vi "Validation Class.vi"() -> ()   [LabVIEW 2020, in "Library Instrument & Equipement.lvlib" / "Library FireBase.lvlib" / "Firebase Recovery_SN.lvclass"]
uses:
  Firebase Recovery_SN.lvclass
  C:/Users/ngarcin/OneDrive - Altyor/Standard TB/Class/Firebase/Source/Firebase Driver/Firebase Driver.lvclass
  Firebase Recovery_SN.lvclass/Firebase Recovery_SN.ctl
panel:
  out "PN":string
  out "Format_SN":string
  out "Incremental_Number":string
  out "sortie d'erreur":errorcluster
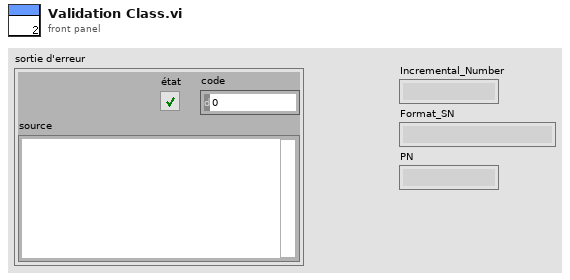
[diagram p1: front panel]
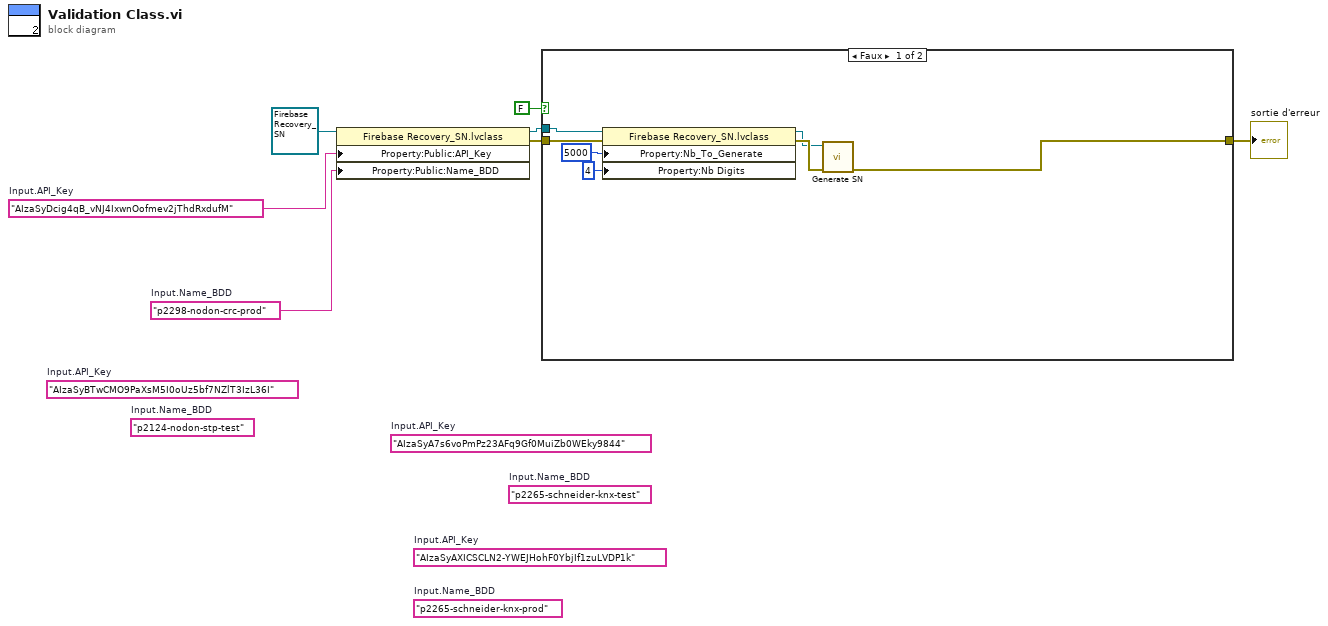
[diagram p0: block diagram]
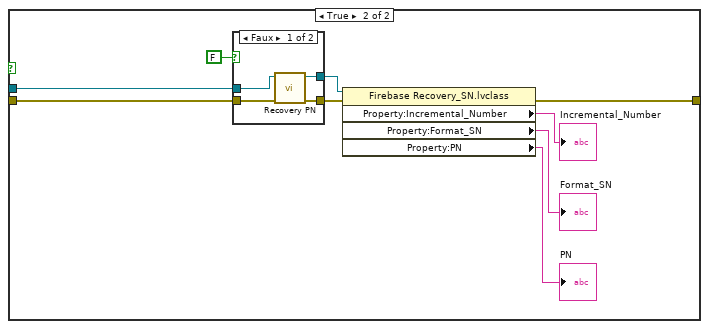
[diagram p2: hidden frame]
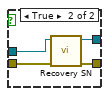
[diagram p3: hidden frame]
diagram:
  (unwired) "AIzaSyBTwCMO9PaXsM5I0oUz5bf7NZlT3IzL36I"  # Input.API_Key
  (unwired) "p2124-nodon-stp-test"  # Input.Name_BDD
  (unwired) "AIzaSyA7s6voPmPz23AFq9Gf0MuiZb0WEky9844"  # Input.API_Key
  (unwired) "p2265-schneider-knx-test"  # Input.Name_BDD
  w2 = "AIzaSyDcig4qB_vNJ4IxwnOofmev2jThdRxdufM"  # Input.API_Key
  w1 = "p2298-nodon-crc-prod"  # Input.Name_BDD
  (unwired) "AIzaSyAXICSCLN2-YWEJHohF0YbjIf1zuLVDP1k"  # Input.API_Key
  (unwired) "p2265-schneider-knx-prod"  # Input.Name_BDD
  n1 = property class="Firebase Recovery_SN.lvclass"(reference=refnum<class "Firebase Recovery_SN.lvclass"> refnum ("Build Library FireBase.lvlib:Firebase AssembledProducts.lvclass"), "Property:Public:API_Key"=w2, "Property:Public:Name_BDD"=w1) -> (reference out=w6:refnum<class "Firebase Recovery_SN.lvclass">, error out=w5:errorcluster)  [unwired: 1 in]
  n2 = case shown="Faux" FALSE {
    tunnel: w6 -> [w11 w23]
    tunnel: w5 -> [w13 w22]
    tunnel: [w14 w19] -> w4
    frame False {
      n3 = property class="Firebase Recovery_SN.lvclass"(reference=w11, error in=w13, "Property:Nb_To_Generate"=u16 5000 ("Nb_To_Generate"), "Property:Nb Digits"=u8 4 ("Nb Digits")) -> (reference out=w10:refnum<class "Firebase Recovery_SN.lvclass">, error out=w12:errorcluster)
      n4 = call-dynamic "Generate SN.vi"("error in (no error)"=w12, "Firebase Recovery_SN en entrée"=w10) -> ("error out"=w14:errorcluster)  [unwired: 8 in, 1 out]
    }
    frame True {
      n5 = case shown="Faux" FALSE {
        tunnel: w23 -> [w27 w31]
        tunnel: w22 -> [w26 w30]
        tunnel: [w25 w29] -> w21
        tunnel: [w24 w28] -> w20
        frame False {
          n6 = call-dynamic "Recovery PN.vi"("error in (no error)"=w26, "Firebase Benches en entrée"=w27) -> ("error out"=w25:errorcluster, "Firebase Benches en sortie"=w24:refnum<class "Firebase Recovery_SN.lvclass">)  [unwired: 8 in]
        }
        frame True {
          n7 = call-dynamic "Recovery SN.vi"("error in (no error)"=w30, "Firebase Benches en entrée"=w31) -> ("error out"=w29:errorcluster, "Firebase Benches en sortie"=w28:refnum<class "Firebase Recovery_SN.lvclass">)  [unwired: 8 in]
        }
      }
      n8 = property class="Firebase Recovery_SN.lvclass"(reference=w20, error in=w21) -> (error out=w19:errorcluster, "Property:Incremental_Number"=→"Incremental_Number":string, "Property:Format_SN"=→"Format_SN":string, "Property:PN"=→"PN":string)  [unwired: 1 out]
    }
  }
  "sortie d'erreur" <- w4
